vi "hidSPD Write Report (poly).vi"   [LabVIEW 2018, in "hidSPDLibForLabView.lvlib"]
uses:
  hidSPDLibForLabView.lvlib
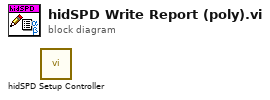
[diagram p0: block diagram]
diagram:
  n1 = call "hidSPD Setup Controller.vi"() -> ()  [unwired: 10 in, 2 out]
